vi "SetGXMLCfgVolt.vi"(8 "error in (no error)":errorcluster, 10 "Voltage Cfg":T1, 11 "Voltage in":refnum<class "Voltage.lvclass">) -> (0 "error out":errorcluster, 3 "Voltage out":refnum<class "Voltage.lvclass">)   [LabVIEW 2012, in "Measurement Channels.lvlib" / "Voltage.lvclass"]
uses:
  Voltage.lvclass
  VoltProps_TD.ctl
  Voltage.lvclass/Voltage.ctl
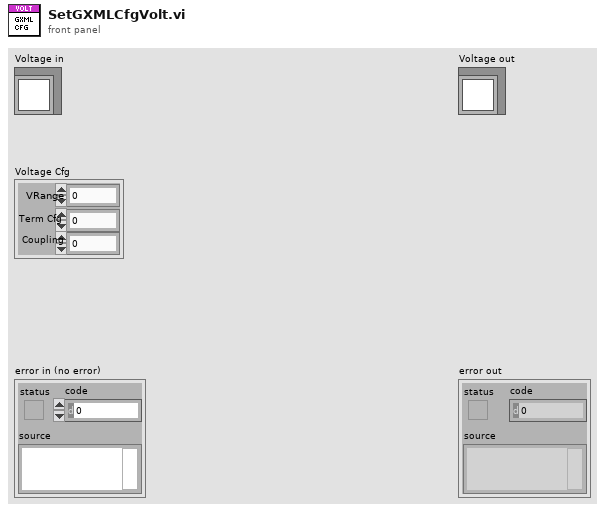
[diagram p1: front panel]
types:
  T1 = typedef "Measurement Channels.lvlib/Voltage.lvclass/VoltProps_TD.ctl" = cluster{"VRange":dbl, "Term Cfg":u16, "Coupling":u16}
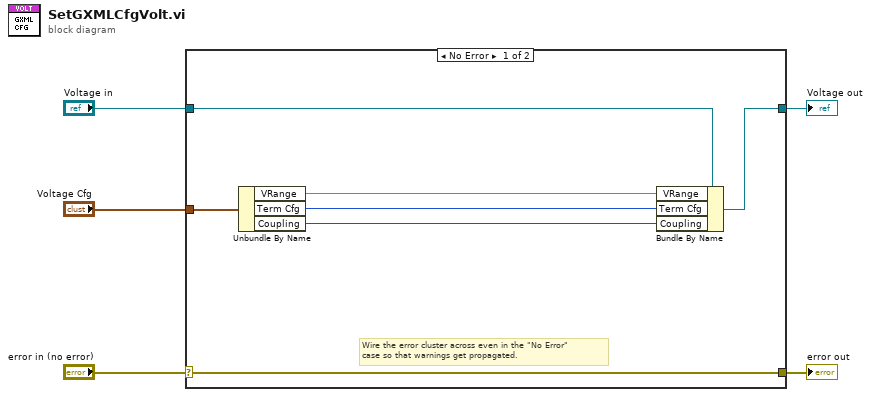
[diagram p0: block diagram]
diagram:
  n1 = case shown="No Error" "error in (no error)" {
    selector: "error in (no error)" -> [w12 w14]
    tunnel: [w12 w14] -> w4
    tunnel: [w6 w13] -> w2
    tunnel: "Voltage in" -> [w9 w13]
    tunnel: "Voltage Cfg" -> [w7 _]
    frame No Error {
      # "Wire the error cluster across even in the \"No Error\"\ncase so that warnings get propagated."
      n2 = Unbundle By Name(w7) -> ("VRange"=w11:dbl, "Term Cfg"=w8:u16, "Coupling"=w10:u16)
      n3 = Bundle By Name(cluster=w9, "VRange"=w11, "Term Cfg"=w8, "Coupling"=w10) -> (w6:refnum<class "Voltage.lvclass">)
    }
    frame Error {
    }
  }
  "error out" <- w4
  "Voltage out" <- w2
